vi "SLSC Convert ENUM Value to ENUM String.vi"(11 "enums":T1[](array[typedef])) -> (3 "string enums":cluster{"name":string, "string enums":string}[](array[cluster]))   [LabVIEW 2017, in "SLSC Tree Control.lvlib"]
doc: "Converts the ENUM datatype into ENUM strings used in the SLSC Output Tree control."
uses:
  SLSC Tree Control.lvlib
  SLSC EDS API/JSON parsing/enum.ctl
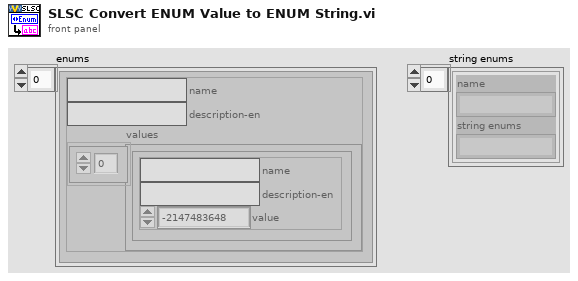
[diagram p1: front panel]
types:
  T1 = typedef "enum.ctl" = cluster{"name":string, "description-en":string, "values":cluster{"name":string, "description-en":string, "value":i32}[]}
  T2 = cluster{"name":string, "description-en":string, "value":i32}[]
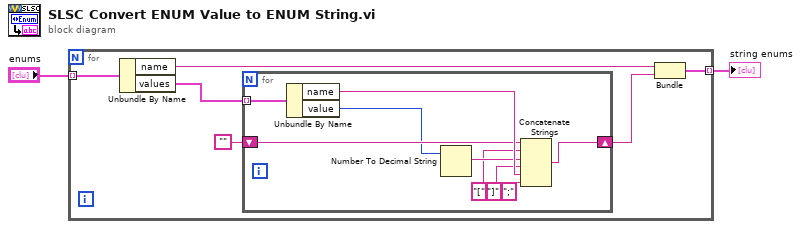
[diagram p0: block diagram]
diagram:
  n1 = for {
    tunnel: "enums" -> [w8] mode=indexing
    tunnel: [w3] -> w2 mode=indexing
    n2 = Unbundle By Name(w8) -> ("name"=w4:string, "values"=w7:T2)
    n3 = for {
      tunnel: w7 -> [w10] mode=indexing
      shift-right: [w16] -> w5
      shift-left: "" -> [w15]
      n4 = Unbundle By Name(w10) -> ("name"=w17:string, "value"=w9:i32)
      n5 = Number To Decimal String(number=w9) -> (decimal integer string=w14:string)  [unwired: 1 in]
      n6 = Concatenate Strings(w15, "[" ("string"), w14, "]" ("string"), w17, ";" ("string")) -> (w16:string)
    }
    n7 = Bundle("name"=w4, w5) -> (w3:cluster{"name":string, string})  [unwired: 1 in]
  }
  "string enums" <- w2
